vi "Write COM Port.vi"(8 "error in (no error)":errorcluster, 10 "COM Port":refnum<visa-resource-name>, 11 "Dimetix Laser in":refnum<class "Dimetix Laser.lvclass">) -> (0 "error out":errorcluster, 3 "Dimetix Laser out":refnum<class "Dimetix Laser.lvclass">)   [LabVIEW 2017, in "Sensors.lvlib" / "Dimetix Laser.lvclass"]
uses:
  Dimetix Laser.lvclass
  Dimetix Laser.lvclass/Dimetix Laser.ctl
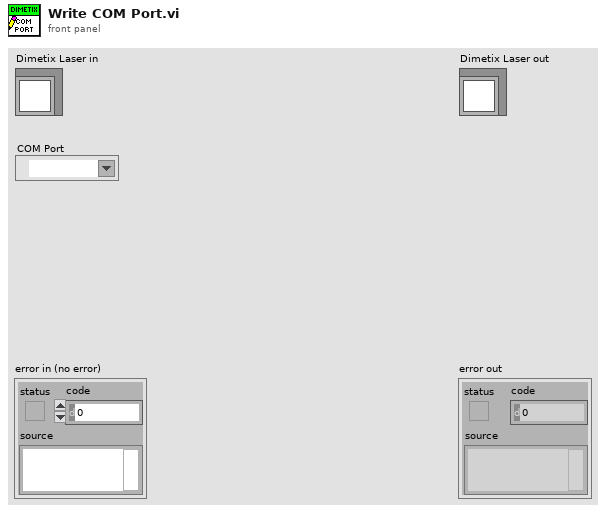
[diagram p1: front panel]
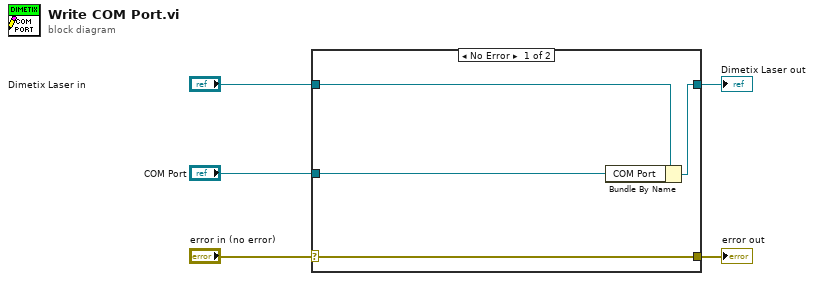
[diagram p0: block diagram]
diagram:
  n1 = case shown="No Error" "error in (no error)" {
    selector: "error in (no error)" -> [w9 w10]
    tunnel: [w9 w10] -> w4
    tunnel: [w7 w11] -> w2
    tunnel: "Dimetix Laser in" -> [w8 w11]
    tunnel: "COM Port" -> [w6 _]
    frame No Error {
      n2 = Bundle By Name(cluster=w8, "COM Port"=w6) -> (w7:refnum<class "Dimetix Laser.lvclass">)
    }
    frame Error {
    }
  }
  "error out" <- w4
  "Dimetix Laser out" <- w2
